vi "DVPW Dynamics Viscosity of Pure Water (Kg to m to s).vi"(1 "Pure Water Temprature":dbl[unit]) -> (0 "DVPW":dbl[unit])   [LabVIEW 2018]
panel:
  out "Pure Water Temprature":dbl[unit](slide) scale=0.0..100.0
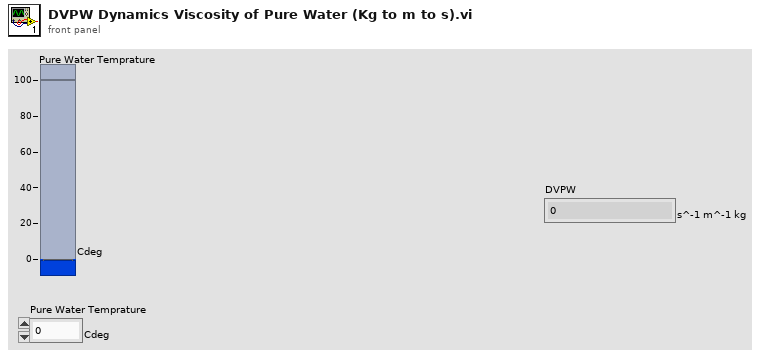
[diagram p1: front panel]
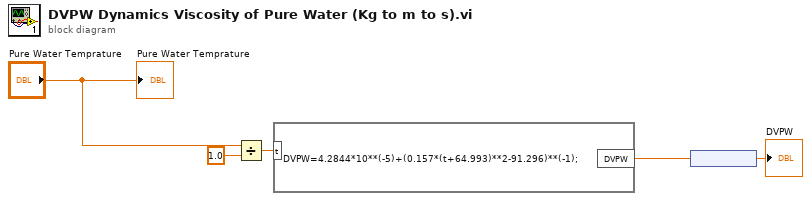
[diagram p0: block diagram]
diagram:
  n1 = Divide(x="Pure Water Temprature", y=dbl[unit] 1.0) -> (x/y=w5:dbl)
  n2 = formula code="DVPW=4.2844*10**(-5)+(0.157*(t+64.993)**2-91.296)**(-1);"("t"=w5) -> ("DVPW"=w1:dbl)
  n3 = node(w1) -> (→"DVPW":dbl[unit])
  "Pure Water Temprature" <- "Pure Water Temprature"
